vi "Receive_Digitals.vi"(0 "Nr of Digitals":u32) -> (1 "Aborted":bool, 2 "Error Out":u8=10)   [LabVIEW 2017]
uses:
  <vilib>/rvi/interface/RandomDataEmulation/niFpgaRandomDataHandleErrors.vi
  <vilib>/rvi/Memory/Memory_Emulation/nirvimemoryFastEmulation.vi
  <vilib>/rvi/Memory/Memory_Emulation/nirvimemoryEmulation.vi
  <vilib>/rvi/Emulation/niFpgaEmulationIsFPGAContextNoSignature.vi
  <vilib>/rvi/DataTransferAndStorage/Container/Common/niFpgaContainerGetUniqueNameForEmu.vi
  <vilib>/rvi/Emulation/niFpgaProcessEmulError.vi
  <vilib>/rvi/Emulation/niFpgaSctlEmulationGetInTimedLoop.vi
  <vilib>/rvi/errors/nirviReportUnexpectedCaseInternalError (U32).vi
  <vilib>/rvi/DataTransferAndStorage/Container/XNode/niFpgaContainer.xnode
  <vilib>/rvi/interface/RandomDataEmulation/nirviRandomDataFpgaReadWriteTemplate.vi
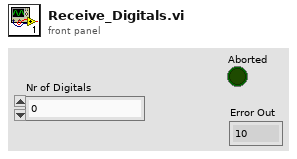
[diagram p1: front panel]
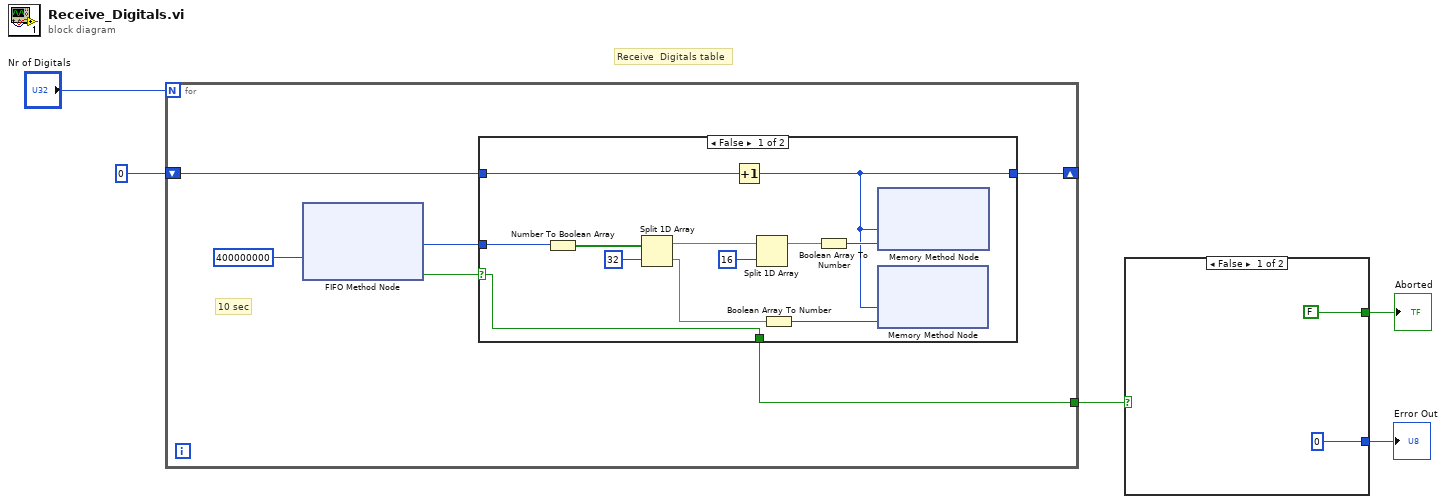
[diagram p0: block diagram]
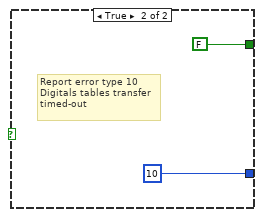
[diagram p3: hidden frame]
diagram:
  # "Receive  Digitals table"
  n1 = for {
    N: "Nr of Digitals" -> [_]
    shift-right: [w7] -> _
    shift-left: u16 0 -> [w8]
    tunnel: [w6] -> w1
    # "10 sec"
    n2 = xnode ("FIFO Method Node")("Timeout"=400000000) -> ("Element"=w10:u64, "Timed Out?"=w9:bool)  [unwired: 1 in, 1 out]
    n3 = case shown="False" w9 {
      selector: w9 -> [w14 w25]
      tunnel: w10 -> [w23 _]
      tunnel: [w14 w25] -> w6
      tunnel: w8 -> [w13 w24]
      tunnel: [w12 w24] -> w7
      frame False {
        n4 = Number To Boolean Array(number=w23) -> (Boolean array=w18:bool[])
        n5 = Split 1D Array(array=w18, index=32) -> (first subarray=w17:bool[], second subarray=w21:bool[])
        n6 = Increment(x=w13) -> (x+1=w12:u16)
        n7 = Split 1D Array(array=w17, index=16) -> (first subarray=w16:bool[])  [unwired: 1 out]
        n8 = Boolean Array To Number(Boolean array=w21) -> (number=w19:u32)
        n9 = Boolean Array To Number(Boolean array=w16) -> (number=w20:u16)
        n10 = xnode ("Memory Method Node")("Address"=w12, "Data"=w20) -> ()  [unwired: 1 in, 1 out]
        n11 = xnode ("Memory Method Node")("Address"=w12, "Data"=w19) -> ()  [unwired: 1 in, 1 out]
      }
      frame True {
      }
    }
  }
  n12 = case shown="False" w1 {
    tunnel: [u8 0 ("Element") u8 10 ("Element")] -> w4
    tunnel: [FALSE FALSE] -> w3
    frame False {
    }
    frame True {
      # "Report error type 10\nDigitals tables transfer \ntimed-out"
    }
  }
  "Error Out" <- w4
  "Aborted" <- w3
